vi "Wire Decode Varint I64.vi"(11 "Buffer in":u8[](array[numeric]) format="%.0x") -> (2 "I64":i64, 3 "Buffer":u8[](array[numeric]) format="%.0x")   [LabVIEW 2020, in "LV-Proto.lvlib"]
uses:
  LV-Proto.lvlib
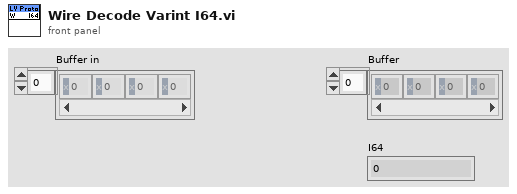
[diagram p1: front panel]
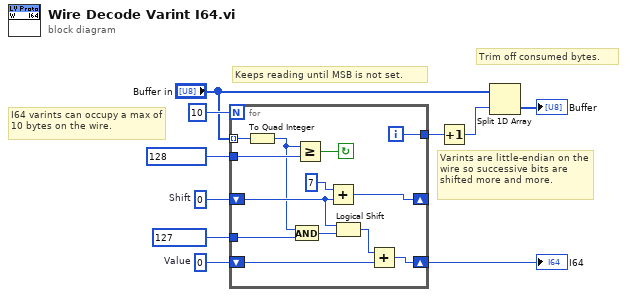
[diagram p0: block diagram]
diagram:
  w7 = 0  # Shift
  w9 = i64 0  # Value
  # "I64 varints can occupy a max of 10 bytes on the wire."
  # "Trim off consumed bytes."
  # "Keeps reading until MSB is not set."
  # "Varints are little-endian on the wire so successive bits are shifted more and more."
  n1 = for {
    N: 10 -> [_]
    shift-right: [w16] -> w6
    shift-left: w9 -> [w17]
    tunnel: "Buffer in" -> [w18] mode=indexing
    tunnel: i64 128 ("y") -> [w23]
    shift-right: [w20] -> _
    shift-left: w7 -> [w19]
    tunnel: [w15] -> w4
    tunnel: i64 127 ("y") -> [w13]
    i -> [w15]
    stop <- w22 continue-if-true
    n2 = To Quad Integer(1:w18) -> (0:w12:i64)
    n3 = And(x=w12, y=w13) -> (x .and. y?=w14:i64)
    n4 = Greater Or Equal?(x=w12, y=w23) -> (x >= y?=w22:bool)
    n5 = Add(x=7, y=w19) -> (x+y=w20:i32)
    n6 = Logical Shift(y=w19, x=w14) -> (x << y=w11:i64)
    n7 = Add(x=w11, y=w17) -> (x+y=w16:i64)
  }
  "I64" <- w6
  n8 = Increment(x=w4) -> (x+1=w1:i32)
  n9 = Split 1D Array(array="Buffer in", index=w1) -> (second subarray=→"Buffer":u8[])  [unwired: 1 out]
